vi "Set Sparse Marker Indexes [SM].vi"(8 "error in (no error)":errorcluster, 9 "Indexes Array":i64[](array[numeric]) caption="indexes array", 10 "Marker Name (\"\")":string caption="marker name (\"\")", 11 "CS++Fgen in":refnum<class "CS++Fgen.lvclass">) -> (0 "error out":errorcluster, 3 "CS++Fgen out":refnum<class "CS++Fgen.lvclass">)   [LabVIEW 2013, in "CS++Fgen.lvlib" / "CS++Fgen.lvclass"]
doc: "The VI sets the indexes associated with the sparse marker. These indexes may be coerced by the driver. Use the IviFgen Get Sparse Marker Indexes [SM] VI to find the coerced values.\n\nNote:\n\n(1) This VI is part of the IviFgenSparseMarker [SM] extension group."
uses:
  CS++Fgen.lvclass
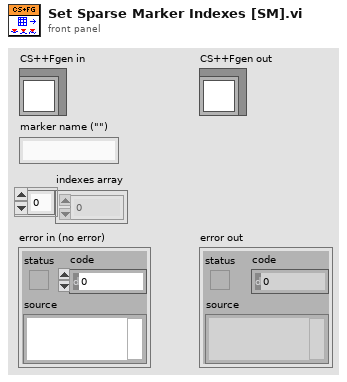
[diagram p1: front panel]
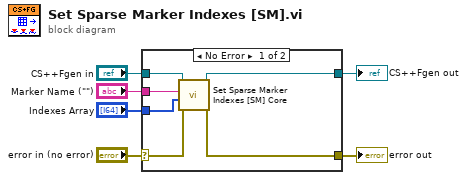
[diagram p0: block diagram]
diagram:
  n1 = case shown="No Error" "error in (no error)" {
    selector: "error in (no error)" -> [w10 w14]
    tunnel: [w9 w14] -> w5
    tunnel: [w11 w13] -> w3
    tunnel: "CS++Fgen in" -> [w12 w13]
    tunnel: "Marker Name (\"\")" -> [w8 _]
    tunnel: "Indexes Array" -> [w7 _]
    frame No Error {
      n2 = call-dynamic "Set Sparse Marker Indexes [SM] Core.vi"("error in (no error)"=w10, "Indexes Array"=w7, "Marker Name (\"\")"=w8, "CS++Fgen in"=w12) -> ("error out"=w9:errorcluster, "CS++Fgen out"=w11:refnum<class "CS++Fgen.lvclass">)  [unwired: 6 in]
    }
    frame Error {
    }
  }
  "error out" <- w5
  "CS++Fgen out" <- w3
